vi "4-bit to num.vi"(1 "Boolean 4":bool, 2 "Boolean 3":bool, 3 "Boolean 2":bool, 4 "Boolean":bool) -> (0 "DIO IN[3:0]":u8)   [LabVIEW 2019]
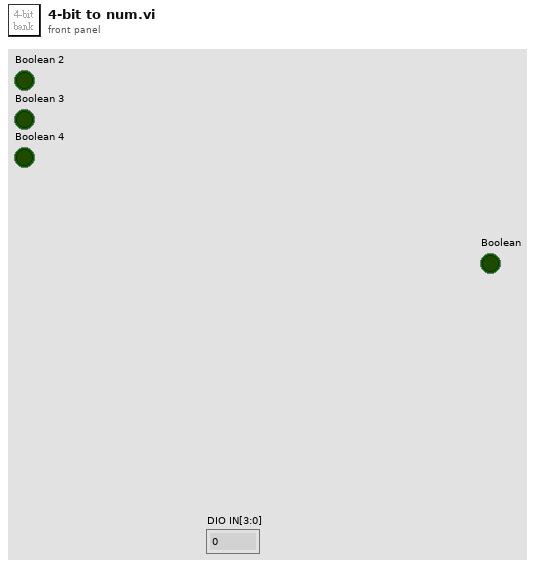
[diagram p1: front panel]
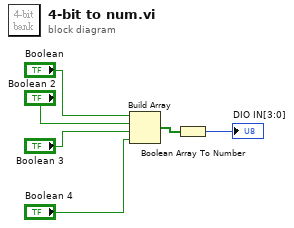
[diagram p0: block diagram]
diagram:
  n1 = Build Array("Boolean", "Boolean 2", "Boolean 3", "Boolean 4") -> (w6:bool[])
  n2 = Boolean Array To Number(Boolean array=w6) -> (number=→"DIO IN[3:0]":u8)
